vi "modbusRTU_v2.vi"() -> ()   [LabVIEW 2019]
uses:
  <vilib>/Modbus/master/Create Master Instance (Serial).vi
  <vilib>/Modbus/master/Modbus Master.lvclass
panel:
  in  "Reset Button":bool
  in  "Limpar":bool
  out "?":T1(graph)
  out "modo (short)":enum16{"short", "long"}(ring) caption="Modo (16 ou 32b)"
  out "sistema 01":enum16{"sistema 01"}(ring) caption="Tipo do sistema"
  out "freq nom":enum16{"50 hz", "60 hz"}(ring) caption="Freq nominal"
  out "formato dado":T2(ring) caption="Formato dado"
  out "polaridade tc":enum16{"(+)", "(-)"}(ring) caption="Polaridade sensor"
  out "Gauge 2 Baud rate":u16(knob) caption="Baud rate" scale=1.0..8.0
  out "Freq instântanea":sgl
  out "Energia ativa total":sgl caption="Energia total kWh" format="%#.4f"
  out "Pot aparente fase A":sgl
  out "Pot reativa fase A":sgl
  out "Pot ativa fase A":sgl
  out "FP fase A":sgl
  out "Corrente fase A":sgl
  out "Tensão fase A":sgl
  out "estado saida IO2":bool caption="Estado saída I/O2"
  in  "holding register value input":u16 caption="Valor\nholding register"
  in  "holding register address":u16(ring) caption="Endereço\nholding register" items=["SPLL"=26, "SPHL"=27, "Type"=43, "Ctrl"=46, "Act"=48, "Atun"=49, "Unit"=67]
  out "SPHL":dbl
  out "SPLL":dbl
  in  "Write Button":bool
  out "Horizontal Pointer Slide Pb":dbl caption="Pb"
  out "Horizontal Pointer Slide Ir":dbl caption="Ir"
  out "Horizontal Pointer Slide 1 Dt":dbl caption="Dt"
  in  "Boolean Run":bool caption="Run"
  out "Gauge Baud rate":u16(knob) caption="Baud rate" scale=0.0..6.0
  in  "exit button":bool
  out "unit ID (nó)":u16 caption="Unit ID (nó)"
  out "Thermometer PV":dbl(slide) caption="PV - Temperatura" scale=0.0..300.0
  out "Unit":enum16{"ºC", "ºF"}(ring)
  out "Atun":T3(ring)
  out "Act":enum16{"rE", "d Ir", ""}(ring)
  out "Run":u16
  out "Ctrl":enum16{"Man", "Auto"}(ring)
  out "Addr (nó)":u16
  out "Type sensor":enum16{"", "tc K"}(ring) caption="Type"
  out "MV":u16(slide) caption="MV \n   ação \n     de \ncontrole" scale=0.0..100.0
  in  "stop button":bool
  in  "start button":bool
  in  "modo Modbus":enum16{"RTU", "ASCII"}(ring)
  in  "VISA resource name \nCOM port":refnum<visa-resource-name>="COM4"
  in  "parity bit":u16(ring)=2 caption="bit de paridade" items=["None", "Odd", "Even"]
  in  "flow control":u16(ring) caption="controle de fluxo" items=["None", "XON/XOFF", "RTS/CTS", "XON/XOFF & RTS/CTS", "DTR/DSR", "XON/XOFF & DTR/DSR"]
  in  "baud rate":u32(ring)=9600 items=["1200"=1200, "2400"=2400, "4800"=4800, "9600"=9600, "19200"=19200, "57600"=57600]
  in  "holding register value SP":u16 caption="Setpoint (SP)"
  # "COMUNICAÇÃO ON/OFF"
  # "CONTROLADOR PID N1200"
  # "MULTIMEDIDOR M-200"
  # "VALORES EM MALHA ABERTA (degrau 220Vca)"
  # "Reading holding \n    registers (03)"
  # "Reading input \n  registers (04)"
  # "167 ºC"
  # "220 Vca"
  # "0,13 A"
  # "FP 0,99"
  # "Writing single \n  registers (06)"
  # "*Valores do sistema sem controle de temperatura"
  # "Reading coils (01)"
  # "MESTRE \nMODBUS  RTU"
  # "Reading holding registers (03)"
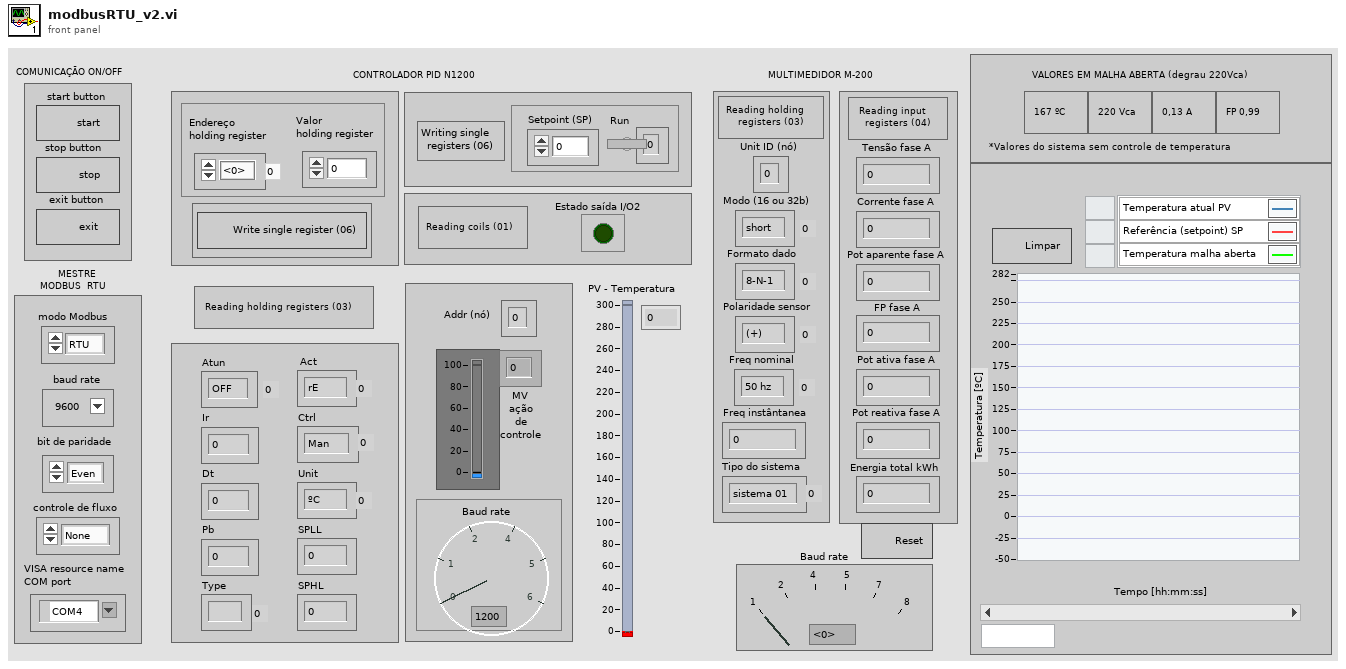
[diagram p1: front panel]
types:
  T1 = cluster{dbl, "y":u16, "holding register value SP":u16}
  T2 = enum16{"8-N-1", "8-N-2", "8-E-1", "8-E-2", "8-O-1", "8-O-2"}
  T3 = enum16{"OFF", "FAST", "FULL", "SELF", "RSELF", "TGHT"}
  T4 = cluster{dbl, "y":u16, "holding register value SP":u16}[]
  T5 = cluster{dbl, "holding register value SP":u16, "y":u16}
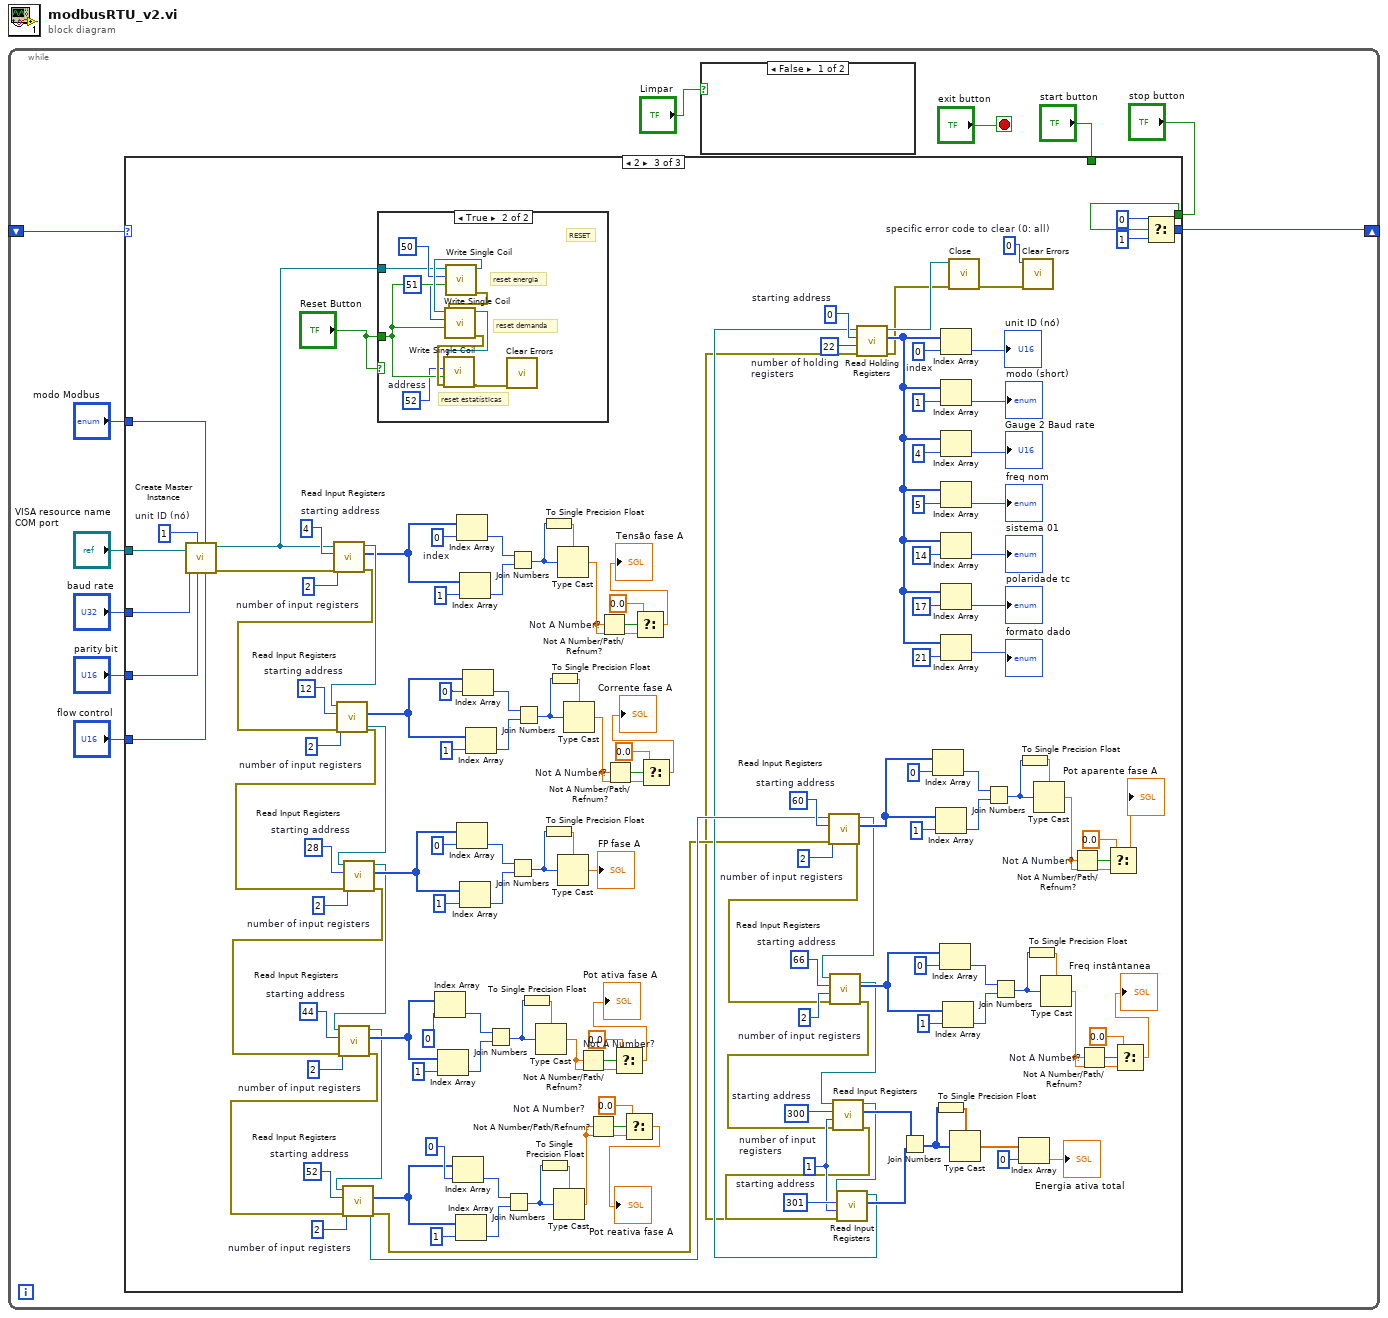
[diagram p0: block diagram]
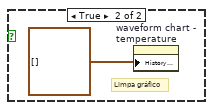
[diagram p2: hidden frame]
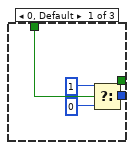
[diagram p3: hidden frame]
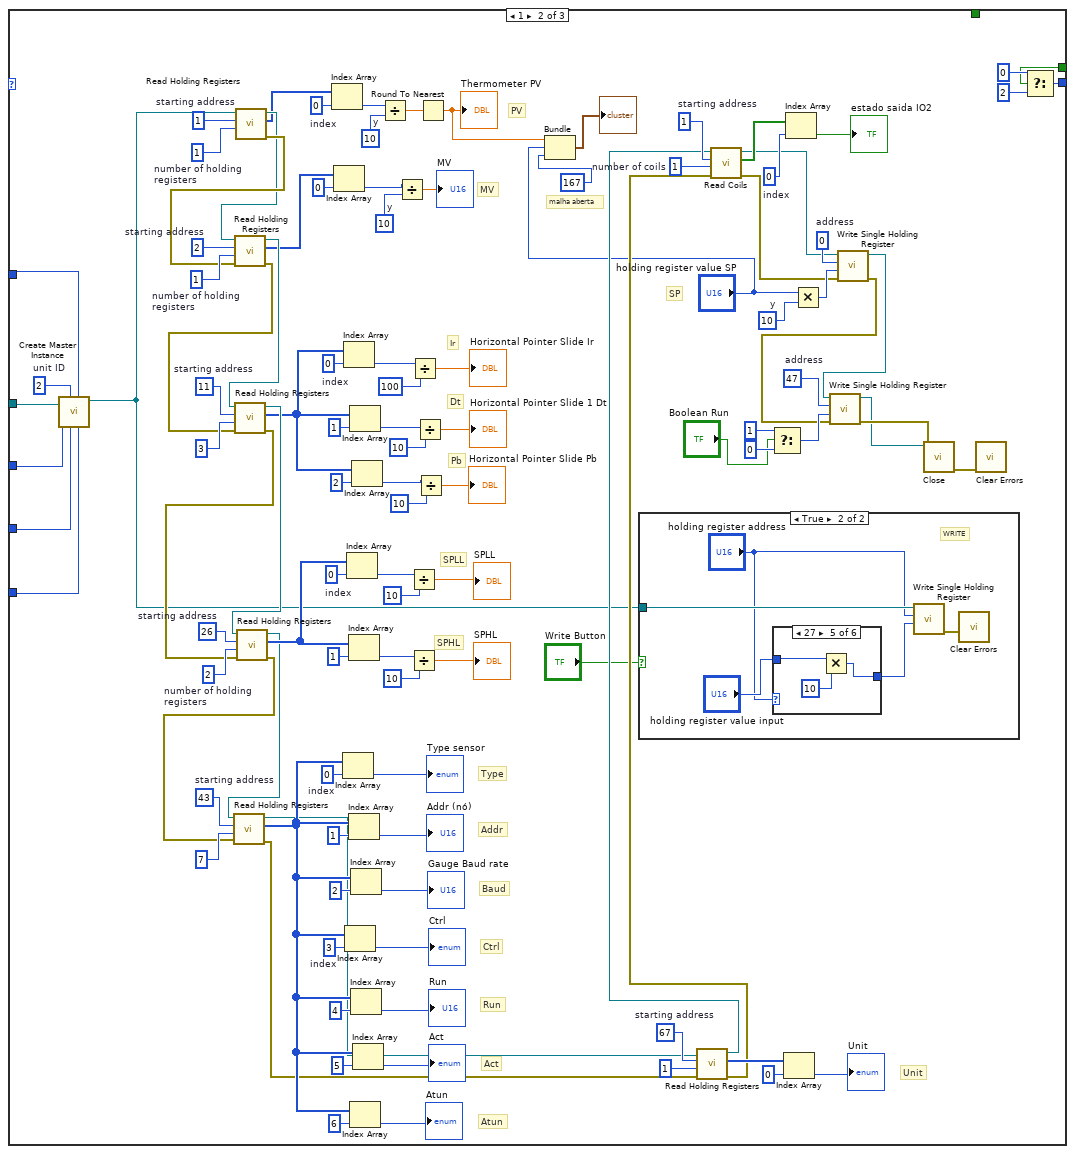
[diagram p4: hidden frame]
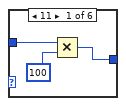
[diagram p6: hidden frame]
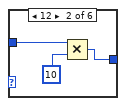
[diagram p7: hidden frame]
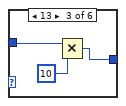
[diagram p8: hidden frame]
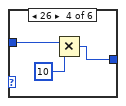
[diagram p9: hidden frame]
diagram:
  n1 = while {
    shift-right: [w10] -> _
    shift-left: _ -> [w11]
    stop <- "exit button" stop-if-true
    n2 = case shown="2" w11 {
      tunnel: [w16 w119 w293] -> w10
      tunnel: "stop button" -> [_ w118 w292]
      tunnel: "modo Modbus" -> [_ w117 w291]
      tunnel: "VISA resource name \nCOM port" -> [_ w116 w290]
      tunnel: "parity bit" -> [_ w114 w289]
      tunnel: "flow control" -> [_ w113 w288]
      tunnel: "baud rate" -> [_ w115 w287]
      tunnel: "start button" -> [w13 _ _]
      frame 0, Default {
        n3 = Select(t=1, s=w13, f=0) -> (s? t:f=w16:i32)
      }
      frame 1 {
        w28 = u16 1  # number of holding registers
        w29 = u16 1  # starting address
        w48 = 0  # index
        w51 = u16 1  # number of coils
        w52 = u16 1  # starting address
        w61 = u16 47  # address
        w65 = u16 10  # y
        w76 = u8 2  # unit ID
        w80 = u16 67  # starting address
        w90 = 3  # index
        w95 = 0  # index
        w97 = u16 43  # starting address
        w101 = 0  # index
        w98 = u16 2  # number of holding registers
        w102 = u16 26  # starting address
        w105 = 0  # index
        w107 = u16 11  # starting address
        w110 = 0  # index
        w111 = u16 10  # y
        w112 = u16 10  # y
        w124 = u16 1  # number of holding registers
        w125 = u16 2  # starting address
        w126 = u16 0  # address
        # "malha aberta"
        # "Unit"
        # "Atun"
        # "Act"
        # "Run"
        # "Ctrl"
        # "Baud"
        # "Addr"
        # "Type"
        # "SPHL"
        # "SPLL"
        # "Pb"
        # "Dt"
        # "Ir"
        # "MV"
        # "PV"
        # "SP"
        n4 = call-poly <vilib>:"Create Master Instance.vi"("flow control (None)"=w113, "serial type"=w117, "parity (Even)"=w114, "unit ID"=w76, "baud rate (9600)"=w115, "VISA resource name"=w116) -> ("serial master instance"=w21:refnum<class "Modbus Master.lvclass">)  [unwired: 4 in, 1 out]
        n5 = call-dynamic "Read Holding Registers.vi"("number of holding registers"=w28, "starting address"=w29, "Modbus master in"=w21) -> ("error out"=w27:errorcluster, "register values"=w22:u16[], "Modbus master out"=w26:refnum<class "Modbus Master.lvclass">)  [unwired: 6 in]
        n6 = call-dynamic "Read Holding Registers.vi"("error in (no error)"=w27, "number of holding registers"=w124, "starting address"=w125, "Modbus master in"=w26) -> ("error out"=w39:errorcluster, "register values"=w23:u16[], "Modbus master out"=w25:refnum<class "Modbus Master.lvclass">)  [unwired: 5 in]
        n7 = call-dynamic "Read Holding Registers.vi"("error in (no error)"=w39, "number of holding registers"=u16 3, "starting address"=w107, "Modbus master in"=w25) -> ("error out"=w38:errorcluster, "register values"=w24:u16[], "Modbus master out"=w45:refnum<class "Modbus Master.lvclass">)  [unwired: 5 in]
        n8 = call-dynamic "Read Holding Registers.vi"("error in (no error)"=w38, "number of holding registers"=w98, "starting address"=w102, "Modbus master in"=w45) -> ("error out"=w37:errorcluster, "register values"=w99:u16[], "Modbus master out"=w44:refnum<class "Modbus Master.lvclass">)  [unwired: 5 in]
        n9 = call-dynamic "Read Holding Registers.vi"("error in (no error)"=w37, "number of holding registers"=u16 7, "starting address"=w97, "Modbus master in"=w44) -> ("error out"=w36:errorcluster, "register values"=w82:u16[], "Modbus master out"=w43:refnum<class "Modbus Master.lvclass">)  [unwired: 5 in]
        n10 = Index Array "Index Array"(array=w22, index=w110) -> (element=w109:u16)
        n11 = Index Array(array=w23, index=0) -> (element=w64:u16)
        n12 = Index Array "Index Array"(array=w82, index=w95) -> (element=→"Type sensor":u16)
        n13 = Index Array "Index Array"(array=w24, index=w105) -> (element=w75:u16)
        n14 = Index Array(array=w82, index=w90) -> (element=→"Ctrl":u16)
        n15 = Index Array "Index Array"(array=w99, index=w101) -> (element=w68:u16)
        n16 = Index Array(array=w99, index=1) -> (element=w66:u16)
        n17 = Index Array(array=w82, index=1) -> (element=→"Addr (nó)":u16)
        n18 = Index Array(array=w24, index=1) -> (element=w72:u16)
        n19 = Index Array(array=w82, index=6) -> (element=→"Atun":u16)
        n20 = Index Array(array=w82, index=2) -> (element=→"Gauge Baud rate":u16)
        n21 = Index Array(array=w82, index=4) -> (element=→"Run":u16)
        n22 = Index Array(array=w24, index=2) -> (element=w70:u16)
        n23 = Index Array(array=w82, index=5) -> (element=→"Act":u16)
        n24 = Divide(x=w109, y=w111) -> (x/y=w122:dbl)
        n25 = Divide(x=w64, y=w65) -> (x/y=→"MV":dbl)
        n26 = Divide(x=w68, y=u16 10) -> (x/y=→"SPLL":dbl)
        n27 = Divide(x=w66, y=u16 10) -> (x/y=→"SPHL":dbl)
        n28 = Divide(x=w75, y=u16 100) -> (x/y=→"Horizontal Pointer Slide Ir":dbl)
        n29 = Divide(x=w72, y=u16 10) -> (x/y=→"Horizontal Pointer Slide 1 Dt":dbl)
        n30 = Divide(x=w70, y=u16 10) -> (x/y=→"Horizontal Pointer Slide Pb":dbl)
        n31 = Round To Nearest(number=w122) -> (nearest integer value=w20:dbl)
        "Thermometer PV" <- w20
        n32 = Bundle(w20, "holding register value SP"="holding register value SP", "y"=u16 167) -> (→"?":T5)  [unwired: 1 in]
        n33 = case shown="True" "Write Button" {
          tunnel: w21 -> [_ w130]
          frame False {
          }
          frame True {
            # "WRITE"
            n34 = case shown="27" "holding register address" {
              tunnel: [w133 w135 w138 w141 w144 w147] -> w129
              tunnel: "holding register value input" -> [w132 w136 w139 w142 w145 w147]
              frame 11 {
                n35 = Multiply(x=w132, y=u16 100) -> (x*y=w133:u16)
              }
              frame 12 {
                n36 = Multiply(x=w136, y=u16 10) -> (x*y=w135:u16)
              }
              frame 13 {
                n37 = Multiply(x=w139, y=u16 10) -> (x*y=w138:u16)
              }
              frame 26 {
                n38 = Multiply(x=w142, y=u16 10) -> (x*y=w141:u16)
              }
              frame 27 {
                n39 = Multiply(x=w145, y=u16 10) -> (x*y=w144:u16)
              }
              frame Default {
              }
            }
            n40 = call-dynamic "Write Single Holding Register.vi"("holding register value"=w129, "address"="holding register address", "Modbus master in"=w130) -> ("error out"=w131:errorcluster)  [unwired: 7 in, 1 out]
            n41 = call <vilib>:"Clear Errors.vi"("error in (no error)"=w131) -> ()  [unwired: 5 in, 2 out]
          }
        }
        n42 = call-dynamic "Read Holding Registers.vi"("error in (no error)"=w36, "number of holding registers"=u16 1, "starting address"=w80, "Modbus master in"=w43) -> ("error out"=w34:errorcluster, "register values"=w78:u16[], "Modbus master out"=w35:refnum<class "Modbus Master.lvclass">)  [unwired: 5 in]
        n43 = call-dynamic "Read Coils.vi"("error in (no error)"=w34, "number of coils"=w51, "starting address"=w52, "Modbus master in"=w35) -> ("error out"=w40:errorcluster, "coil values"=w49:bool[], "Modbus master out"=w46:refnum<class "Modbus Master.lvclass">)  [unwired: 5 in]
        n44 = Select(t=u16 1, s="Boolean Run", f=u16 0) -> (s? t:f=w58:u16)
        n45 = Index Array(array=w78, index=0) -> (element=→"Unit":u16)
        n46 = Index Array "Index Array"(array=w49, index=w48) -> (element=→"estado saida IO2":bool)
        n47 = Multiply(x="holding register value SP", y=w112) -> (x*y=w123:u16)
        n48 = call-dynamic "Write Single Holding Register.vi"("error in (no error)"=w40, "holding register value"=w123, "address"=w126, "Modbus master in"=w46) -> ("error out"=w41:errorcluster, "Modbus master out"=w50:refnum<class "Modbus Master.lvclass">)  [unwired: 6 in]
        n49 = call-dynamic "Write Single Holding Register.vi"("error in (no error)"=w41, "holding register value"=w58, "address"=w61, "Modbus master in"=w50) -> ("error out"=w33:errorcluster, "Modbus master out"=w32:refnum<class "Modbus Master.lvclass">)  [unwired: 6 in]
        n50 = call-dynamic "Close.vi"("error in (no error)"=w33, "Modbus master in"=w32) -> ("error out"=w42:errorcluster)  [unwired: 9 in]
        n51 = call <vilib>:"Clear Errors.vi"("error in (no error)"=w42) -> ()  [unwired: 5 in, 2 out]
        n52 = Select(t=0, s=w118, f=2) -> (s? t:f=w119:i32)
      }
      frame 2 {
        w180 = 0  # specific error code to clear (0: all)
        w212 = u16 2  # number of input registers
        w213 = u16 66  # starting address
        w218 = u16 2  # number of input registers
        w219 = u16 60  # starting address
        w220 = u16 2  # number of input registers
        w221 = u16 52  # starting address
        w222 = u16 2  # number of input registers
        w223 = u16 44  # starting address
        w224 = u16 2  # number of input registers
        w225 = u16 28  # starting address
        w226 = u16 2  # number of input registers
        w227 = u16 12  # starting address
        w236 = u16 301  # starting address
        w237 = u16 300  # starting address
        w228 = u16 1  # number of input registers
        w272 = 0  # index
        w275 = u16 2  # number of input registers
        w276 = u16 4  # starting address
        w284 = u8 1  # unit ID (nó)
        w286 = 0  # index
        w297 = u16 0  # starting address
        w296 = u16 22  # number of holding registers
        n53 = call-poly <vilib>:"Create Master Instance.vi"("flow control (None)"=w288, "serial type"=w291, "parity (Even)"=w289, "unit ID"=w284, "baud rate (9600)"=w287, "VISA resource name"=w290) -> ("error out"=w192:errorcluster, "serial master instance"=w148:refnum<class "Modbus Master.lvclass">)  [unwired: 4 in]
        n54 = call-dynamic "Read Input Registers.vi"("error in (no error)"=w192, "number of input registers"=w275, "starting address"=w276, "Modbus master in"=w148) -> ("error out"=w191:errorcluster, "register values"=w215:u16[], "Modbus master out"=w217:refnum<class "Modbus Master.lvclass">)  [unwired: 5 in]
        n55 = call-dynamic "Read Input Registers.vi"("error in (no error)"=w191, "number of input registers"=w226, "starting address"=w227, "Modbus master in"=w217) -> ("error out"=w190:errorcluster, "register values"=w202:u16[], "Modbus master out"=w216:refnum<class "Modbus Master.lvclass">)  [unwired: 5 in]
        n56 = call-dynamic "Read Input Registers.vi"("error in (no error)"=w190, "number of input registers"=w224, "starting address"=w225, "Modbus master in"=w216) -> ("error out"=w189:errorcluster, "register values"=w203:u16[], "Modbus master out"=w200:refnum<class "Modbus Master.lvclass">)  [unwired: 5 in]
        n57 = call-dynamic "Read Input Registers.vi"("error in (no error)"=w189, "number of input registers"=w222, "starting address"=w223, "Modbus master in"=w200) -> ("error out"=w188:errorcluster, "register values"=w204:u16[], "Modbus master out"=w199:refnum<class "Modbus Master.lvclass">)  [unwired: 5 in]
        n58 = call-dynamic "Read Input Registers.vi"("error in (no error)"=w188, "number of input registers"=w220, "starting address"=w221, "Modbus master in"=w199) -> ("error out"=w187:errorcluster, "register values"=w201:u16[], "Modbus master out"=w198:refnum<class "Modbus Master.lvclass">)  [unwired: 5 in]
        n59 = case shown="True" "Reset Button" {
          tunnel: "Reset Button" -> [_ w302]
          tunnel: w148 -> [_ w298]
          frame False {
          }
          frame True {
            w301 = u16 52  # address
            # "RESET"
            # "reset estatísticas"
            # "reset demanda"
            # "reset energia"
            n60 = call-dynamic "Write Single Coil.vi"("coil value"=w302, "address"=u16 50, "Modbus master in"=w298) -> ("error out"=w307:errorcluster, "Modbus master out"=w304:refnum<class "Modbus Master.lvclass">)  [unwired: 7 in]
            n61 = call-dynamic "Write Single Coil.vi"("error in (no error)"=w307, "coil value"=w302, "address"=u16 51, "Modbus master in"=w304) -> ("error out"=w306:errorcluster, "Modbus master out"=w303:refnum<class "Modbus Master.lvclass">)  [unwired: 6 in]
            n62 = call-dynamic "Write Single Coil.vi"("error in (no error)"=w306, "coil value"=w302, "address"=w301, "Modbus master in"=w303) -> ("error out"=w305:errorcluster)  [unwired: 6 in, 1 out]
            n63 = call <vilib>:"Clear Errors.vi"("error in (no error)"=w305) -> ()  [unwired: 5 in, 2 out]
          }
        }
        n64 = Index Array(array=w204, index=0) -> (element=w252:u16)
        n65 = Index Array(array=w204, index=1) -> (element=w250:u16)
        n66 = Index Array(array=w201, index=0) -> (element=w246:u16)
        n67 = Index Array(array=w201, index=1) -> (element=w244:u16)
        n68 = Index Array "Index Array"(array=w215, index=w272) -> (element=w271:u16)
        n69 = Index Array(array=w203, index=0) -> (element=w259:u16)
        n70 = Index Array(array=w215, index=1) -> (element=w269:u16)
        n71 = Index Array(array=w203, index=1) -> (element=w257:u16)
        n72 = Index Array(array=w202, index=0) -> (element=w265:u16)
        n73 = Index Array(array=w202, index=1) -> (element=w263:u16)
        n74 = Join Numbers(hi=w252, lo=w250) -> ((hi.lo)=w254:u32)
        n75 = Join Numbers(hi=w246, lo=w244) -> ((hi.lo)=w248:u32)
        n76 = Join Numbers(hi=w271, lo=w269) -> ((hi.lo)=w273:u32)
        n77 = Join Numbers(hi=w259, lo=w257) -> ((hi.lo)=w261:u32)
        n78 = Join Numbers(hi=w265, lo=w263) -> ((hi.lo)=w267:u32)
        n79 = To Single Precision Float(number=w254) -> (single precision float=w255:sgl)
        n80 = Type Cast(type=w255, x=w254) -> (*(type *) &x=w163:sgl)
        n81 = To Single Precision Float(number=w248) -> (single precision float=w249:sgl)
        n82 = To Single Precision Float(number=w273) -> (single precision float=w274:sgl)
        n83 = To Single Precision Float(number=w261) -> (single precision float=w262:sgl)
        n84 = To Single Precision Float(number=w267) -> (single precision float=w268:sgl)
        n85 = Type Cast(type=w249, x=w248) -> (*(type *) &x=w158:sgl)
        n86 = Type Cast(type=w274, x=w273) -> (*(type *) &x=w171:sgl)
        n87 = Type Cast(type=w262, x=w261) -> (*(type *) &x=→"FP fase A":sgl)
        n88 = Type Cast(type=w268, x=w267) -> (*(type *) &x=w167:sgl)
        n89 = Not A Number/Path/Refnum? "Not A Number?"(number/path/refnum=w163) -> (NaN/Path/Refnum?=w165:bool)
        n90 = Not A Number/Path/Refnum? "Not A Number?"(number/path/refnum=w158) -> (NaN/Path/Refnum?=w161:bool)
        n91 = Not A Number/Path/Refnum? "Not A Number?"(number/path/refnum=w171) -> (NaN/Path/Refnum?=w173:bool)
        n92 = Not A Number/Path/Refnum? "Not A Number?"(number/path/refnum=w167) -> (NaN/Path/Refnum?=w169:bool)
        n93 = Select(t=0.0, s=w165, f=w163) -> (s? t:f=→"Pot ativa fase A":dbl)
        n94 = Select(t=0.0, s=w161, f=w158) -> (s? t:f=→"Pot reativa fase A":dbl)
        n95 = Select(t=0.0, s=w173, f=w171) -> (s? t:f=→"Tensão fase A":dbl)
        n96 = Select(t=0.0, s=w169, f=w167) -> (s? t:f=→"Corrente fase A":dbl)
        n97 = call-dynamic "Read Input Registers.vi"("error in (no error)"=w187, "number of input registers"=w218, "starting address"=w219, "Modbus master in"=w198) -> ("error out"=w186:errorcluster, "register values"=w214:u16[], "Modbus master out"=w197:refnum<class "Modbus Master.lvclass">)  [unwired: 5 in]
        n98 = call-dynamic "Read Input Registers.vi"("error in (no error)"=w186, "number of input registers"=w212, "starting address"=w213, "Modbus master in"=w197) -> ("error out"=w185:errorcluster, "register values"=w205:u16[], "Modbus master out"=w196:refnum<class "Modbus Master.lvclass">)  [unwired: 5 in]
        n99 = call-dynamic "Read Input Registers.vi"("error in (no error)"=w185, "number of input registers"=w228, "starting address"=w237, "Modbus master in"=w196) -> ("error out"=w184:errorcluster, "register values"=w235:u16[], "Modbus master out"=w195:refnum<class "Modbus Master.lvclass">)  [unwired: 5 in]
        n100 = call-dynamic "Read Input Registers.vi"("error in (no error)"=w184, "number of input registers"=w228, "starting address"=w236, "Modbus master in"=w195) -> ("error out"=w183:errorcluster, "register values"=w234:u16[], "Modbus master out"=w194:refnum<class "Modbus Master.lvclass">)  [unwired: 5 in]
        n101 = call-dynamic "Read Holding Registers.vi"("error in (no error)"=w183, "number of holding registers"=w296, "starting address"=w297, "Modbus master in"=w194) -> ("error out"=w182:errorcluster, "register values"=w277:u16[], "Modbus master out"=w193:refnum<class "Modbus Master.lvclass">)  [unwired: 5 in]
        n102 = Join Numbers(hi=w235, lo=w234) -> ((hi.lo)=w232:u32[])
        n103 = Index Array(array=w214, index=0) -> (element=w240:u16)
        n104 = Index Array(array=w214, index=1) -> (element=w238:u16)
        n105 = To Single Precision Float(number=w232) -> (single precision float=w233:sgl[])
        n106 = Index Array(array=w205, index=0) -> (element=w208:u16)
        n107 = Index Array "Index Array"(array=w277, index=w286) -> (element=→"unit ID (nó)":u16)
        n108 = Index Array(array=w277, index=1) -> (element=→"modo (short)":u16)
        n109 = Index Array(array=w277, index=4) -> (element=→"Gauge 2 Baud rate":u16)
        n110 = Index Array(array=w277, index=5) -> (element=→"freq nom":u16)
        n111 = Index Array(array=w277, index=14) -> (element=→"sistema 01":u16)
        n112 = Index Array(array=w277, index=17) -> (element=→"polaridade tc":u16)
        n113 = Index Array(array=w277, index=21) -> (element=→"formato dado":u16)
        n114 = Index Array(array=w205, index=1) -> (element=w206:u16)
        n115 = call-dynamic "Close.vi"("error in (no error)"=w182, "Modbus master in"=w193) -> ("error out"=w181:errorcluster)  [unwired: 9 in]
        n116 = Type Cast(type=w233, x=w232) -> (*(type *) &x=w231:sgl[])
        n117 = Join Numbers(hi=w240, lo=w238) -> ((hi.lo)=w242:u32)
        n118 = Join Numbers(hi=w208, lo=w206) -> ((hi.lo)=w210:u32)
        n119 = Index Array(array=w231, index=0) -> (element=→"Energia ativa total":sgl)
        n120 = To Single Precision Float(number=w242) -> (single precision float=w243:sgl)
        n121 = call <vilib>:"Clear Errors.vi"("error in (no error)"=w181, "specific error code to clear (0: all)"=w180) -> ()  [unwired: 4 in, 2 out]
        n122 = To Single Precision Float(number=w210) -> (single precision float=w211:sgl)
        n123 = Type Cast(type=w243, x=w242) -> (*(type *) &x=w150:sgl)
        n124 = Type Cast(type=w211, x=w210) -> (*(type *) &x=w154:sgl)
        n125 = Not A Number/Path/Refnum? "Not A Number?"(number/path/refnum=w150) -> (NaN/Path/Refnum?=w153:bool)
        n126 = Not A Number/Path/Refnum? "Not A Number?"(number/path/refnum=w154) -> (NaN/Path/Refnum?=w157:bool)
        n127 = Select(t=0.0, s=w153, f=w150) -> (s? t:f=→"Pot aparente fase A":dbl)
        n128 = Select(t=0.0, s=w157, f=w154) -> (s? t:f=→"Freq instântanea":dbl)
        n129 = Select(t=0, s=w292, f=1) -> (s? t:f=w293:i32)
      }
    }
    n130 = case shown="False" "Limpar" {
      frame False {
      }
      frame True {
        # "Limpa gráfico"
        n131 = property on="waveform chart - temperature" class="WFChart (strict)"("History Data"=T4 []) -> ()  [unwired: 2 in, 2 out]
      }
    }
  }
